vi "Digital Pattern Page.vi"(8 "error in (no error)":errorcluster, 11 "Node Ptr":T1 format="%.0x") -> (0 "error out":errorcluster)   [LabVIEW 2017, in "Engine Simulation Toolkit System Explorer.lvlib"]
uses:
  Engine Simulation Toolkit System Explorer.lvlib
  <vilib>/NI Veristand/Custom Device API/Custom Device Item Ref.ctl
  Shared/Properties.vi
  <vilib>/NI Veristand/Custom Device API/Get Item Property (String).vi
  <vilib>/NI Veristand/Custom Device API/Custom Device API.lvlib
  Shared/Engine Simulation Toolkit Shared.lvlib
panel:
  out "Name in bitfile":string
  in  "Name":string
  in  "Header":cluster{"Section Name":string}={"Section Name"="Digital Pattern"}
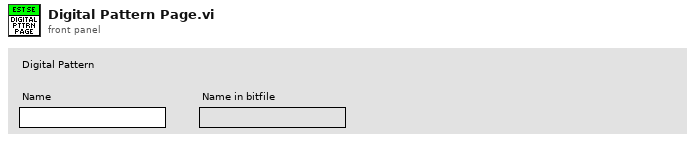
[diagram p1: front panel]
types:
  T1 = typedef "Custom Device API.lvlib/Custom Device Item Ref.ctl" = u64
  T2 = typedef "Custom Device API.lvlib/Custom Device Item Info.ctl" = cluster{"Name":string, "Is Channel":bool, "GUID":string, "Is Waveform":bool}
  T3 = typedef "Custom Device API.lvlib/Custom Device Commands.ctl" = enum16{"Default", "Item renamed", "Shutdown", "Dynamic button pressed"}
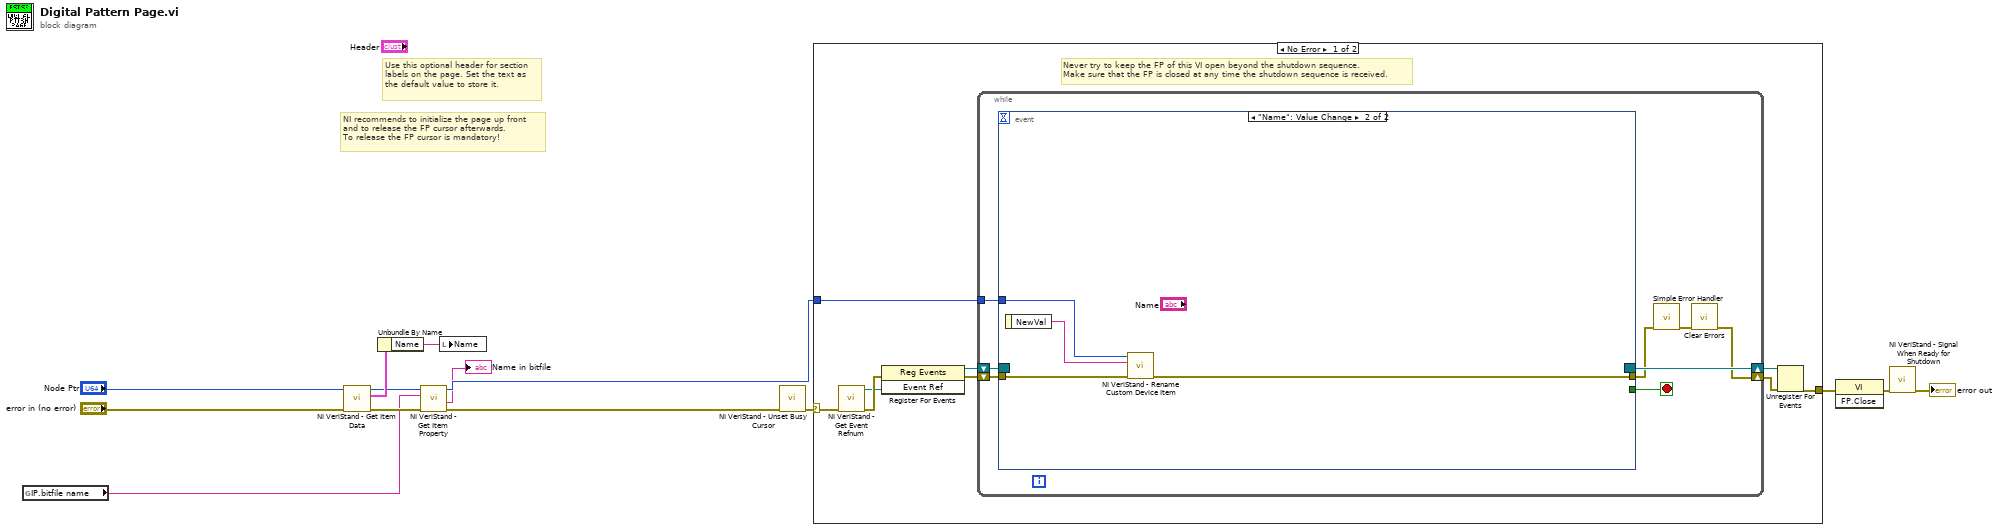
[diagram p0: block diagram]
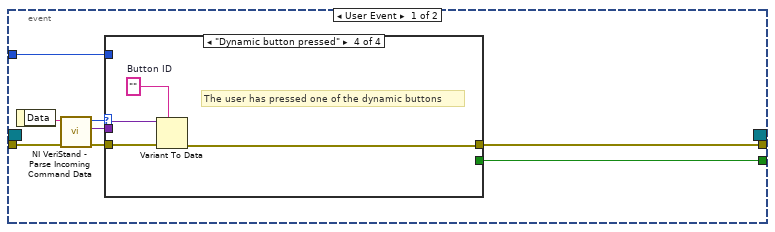
[diagram p2: hidden frame]
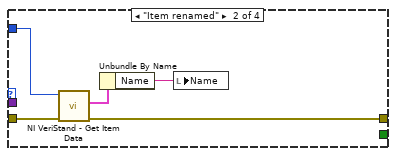
[diagram p4: hidden frame]
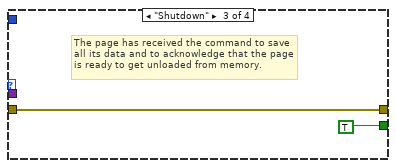
[diagram p5: hidden frame]
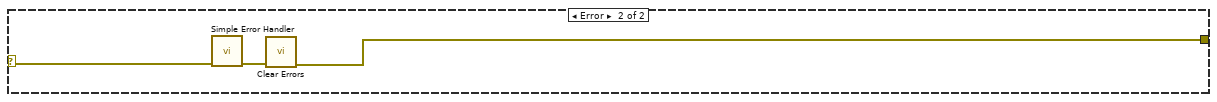
[diagram p6: hidden frame]
diagram:
  # "Use this optional header for section labels on the page. Set the text as the default value to store it."
  # "NI recommends to initialize the page up front\nand to release the FP cursor afterwards.\nTo release the FP cursor is mandatory!"
  n1 = global read "Properties.vi" "IP.bitfile name"() -> (w2:string)
  n2 = call <vilib>:"NI VeriStand - Get Item Data.vi"("error in (no error)"="error in (no error)", "Item Ref in"="Node Ptr") -> ("error out"=w8:errorcluster, "Item Info"=w7:T2, "Item Ref out"=w4:T1)  [unwired: 6 in, 1 out]
  n3 = Unbundle By Name(w7) -> ("Name"=w6:string)
  n4 = call-poly <vilib>:"NI VeriStand - Get Item Property.vi"("error in (no error)"=w8, "Property Name"=w2, "Item Ref in"=w4) -> ("error out"=w5:errorcluster, "Value"=→"Name in bitfile":string, "Item Ref out"=w3:T1)  [unwired: 5 in, 1 out]
  n5 = local write "Name"(w6) -> ()
  n6 = call <vilib>:"NI VeriStand - Unset Busy Cursor.vi"("error in (no error)"=w5) -> ("error out"=w10:errorcluster)  [unwired: 10 out]
  n7 = case shown="No Error" w10 {
    selector: w10 -> [w15 w58]
    tunnel: [w20 w56] -> w14
    tunnel: w3 -> [w16 _]
    frame No Error {
      # "Never try to keep the FP of this VI open beyond the shutdown sequence.\nMake sure that the FP is closed at any time the shutdown sequence is received."
      n8 = call <vilib>:"NI VeriStand - Get Event Refnum.vi"("error in (no error)"=w15) -> ("error out"=w23:errorcluster, "Event Ref"=w19:refnum<user-event>)  [unwired: 9 out]
      n9 = register-events(error in=w23, w19) -> (reference out=w17:refnum<event-registration>, error out=w18:errorcluster)  [unwired: 1 in]
      n10 = while {
        tunnel: w16 -> [w27]
        shift-right: [w24] -> w21
        shift-left: w18 -> [w30]
        shift-right: [w31] -> w22
        shift-left: w17 -> [w29]
        stop <- w28 stop-if-true
        n11 = event shown="[1] \"Name\": Value Change" {
          selector: w29 -> [_ _]
          dyn-events: [_ _] -> w31
          timeout: _ -> [_ _]
          tunnel: w30 -> [w39 w55]
          tunnel: [w35 _] -> w28
          tunnel: [w34 w54] -> w26
          tunnel: w27 -> [w33 w53]
          event User Event {
            n12 = event-data() -> ("Data"=w38:string)  [unwired: 1 out]
            n13 = call <vilib>:"NI VeriStand - Parse Incoming Command Data.vi"("error in (no error)"=w39, "Incoming data"=w38) -> ("error out"=w37:errorcluster, "Outgoing data"=w32:variant, "Action"=w36:T3)  [unwired: 7 out]
            n14 = case shown="\"Dynamic button pressed\"" w36 {
              tunnel: w37 -> [w40 w45 w46 w51]
              tunnel: [_ _ TRUE _] -> w35
              tunnel: [w40 w41 w46 w48] -> w34
              tunnel: w33 -> [_ w44 _ _]
              tunnel: w32 -> [_ _ _ w50]
              frame "Default", Default {
              }
              frame "Item renamed" {
                n15 = call <vilib>:"NI VeriStand - Get Item Data.vi"("error in (no error)"=w45, "Item Ref in"=w44) -> ("error out"=w41:errorcluster, "Item Info"=w42:T2)  [unwired: 6 in, 2 out]
                n16 = Unbundle By Name(w42) -> ("Name"=w43:string)
                n17 = local write "Name"(w43) -> ()
              }
              frame "Shutdown" {
                # "The page has received the command to save all its data and to acknowledge that the page is ready to get unloaded from memory."
              }
              frame "Dynamic button pressed" {
                w49 = ""  # Button ID
                # "The user has pressed one of the dynamic buttons"
                n18 = Variant To Data(error in=w51, type=w49, Variant=w50) -> (error out=w48:errorcluster)  [unwired: 1 out]
              }
            }
          }
          event "Name": Value Change {
            n19 = event-data() -> ("NewVal"=w52:string)  [unwired: 1 out]
            n20 = call <vilib>:"NI VeriStand - Rename Custom Device Item.vi"("error in (no error)"=w55, "New Name"=w52, "Item Ref in"=w53) -> ("error out"=w54:errorcluster)  [unwired: 6 in, 2 out]
          }
        }
        n21 = call <vilib>:"Simple Error Handler.vi"("error in (no error)"=w26) -> ("error out"=w25:errorcluster)  [unwired: 1 in, 7 out]
        n22 = call <vilib>:"Clear Errors.vi"("error in (no error)"=w25) -> ("error out"=w24:errorcluster)  [unwired: 1 in, 5 out]
      }
      n23 = Unregister For Events(event registration refnum=w22, error in=w21) -> (error out=w20:errorcluster)
    }
    frame Error {
      n24 = call <vilib>:"Simple Error Handler.vi"("error in (no error)"=w58) -> ("error out"=w57:errorcluster)  [unwired: 1 in, 7 out]
      n25 = call <vilib>:"Clear Errors.vi"("error in (no error)"=w57) -> ("error out"=w56:errorcluster)  [unwired: 1 in, 5 out]
    }
  }
  n26 = invoke class="VI" method="FP.Close"(error in=w14) -> (error out=w13:errorcluster)  [unwired: 2 in, 2 out]
  n27 = call <vilib>:"NI VeriStand - Signal When Ready for Shutdown.vi"("error in (no error)"=w13) -> ("error out"=→"error out":errorcluster)  [unwired: 10 out]
